vi "Delete Recipe.vi"(8 "error in (no error)":errorcluster, 9 "Delete Row":u16, 11 "MASTER in":refnum<class "MASTER.lvclass">) -> (0 "error out":errorcluster, 3 "MASTER out":refnum<class "MASTER.lvclass">)   [LabVIEW 2014, in "Files Library.lvlib" / "MASTER.lvclass"]
uses:
  MASTER/MASTER.lvclass
  MASTER/MASTER.lvclass/MASTER.ctl
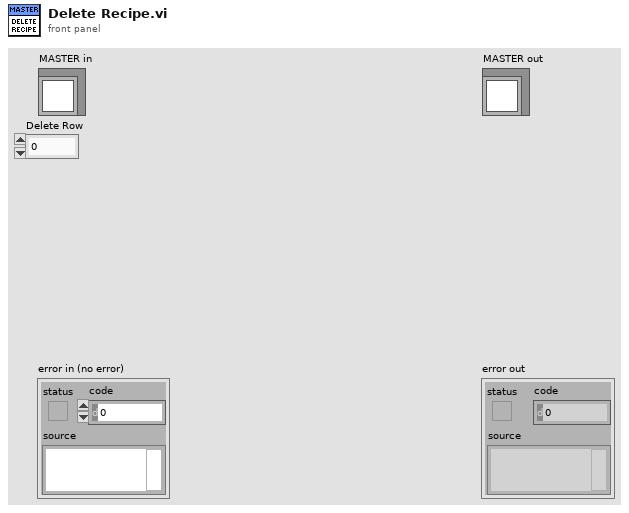
[diagram p1: front panel]
types:
  T1 = typedef "Recipes Indicators.ctl" = cluster{"Speed":string, "Temperature SP":string, "Time Limit":string, "Direction":string}
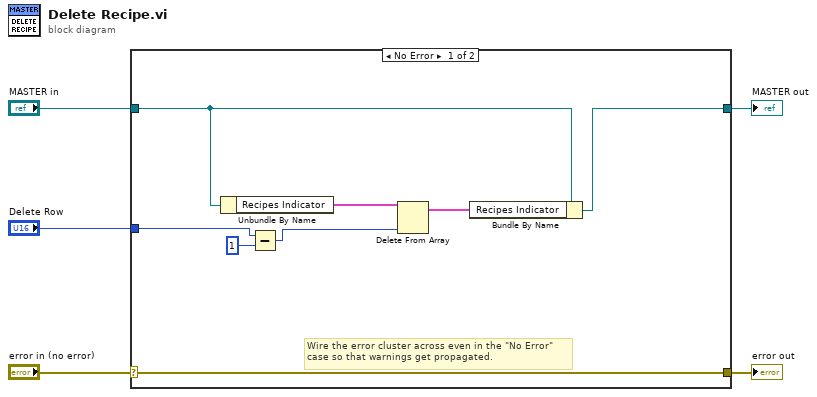
[diagram p0: block diagram]
diagram:
  n1 = case shown="No Error" "error in (no error)" {
    selector: "error in (no error)" -> [w13 w15]
    tunnel: [w13 w15] -> w4
    tunnel: [w9 w14] -> w2
    tunnel: "MASTER in" -> [w10 w14]
    tunnel: "Delete Row" -> [w7 _]
    frame No Error {
      # "Wire the error cluster across even in the \"No Error\"\ncase so that warnings get propagated."
      n2 = Unbundle By Name(w10) -> ("Recipes Indicator"=w12:T1[])
      n3 = Subtract(x=w7, y=u16 1) -> (x-y=w8:u16)
      n4 = Delete From Array(array=w12, index=w8) -> (array with subset deleted=w11:T1[])  [unwired: 1 in, 1 out]
      n5 = Bundle By Name(cluster=w10, "Recipes Indicator"=w11) -> (w9:refnum<class "MASTER.lvclass">)
    }
    frame Error {
    }
  }
  "error out" <- w4
  "MASTER out" <- w2
